vi "TX-SIS-SIM-UDP (SubVI).vi"(5 "SIS-10SDV502":bool, 6 "error in (no error)":errorcluster, 7 "SIS-10SDV501":bool, 8 "UDP Network Connection in":refnum<k16>, 9 "SIM-PC-IP":u32, 10 "SIM-PC-UDP-Port":u16, 11 "SIS-10SDV500":bool) -> (0 "UDP Network Connection out":refnum<k16>, 3 "BPCS-SIM-TX-ARRAY":i16[](array[numeric]), 4 "error out":errorcluster)   [LabVIEW 2018]
panel:
  out "length":i32[](array[numeric])
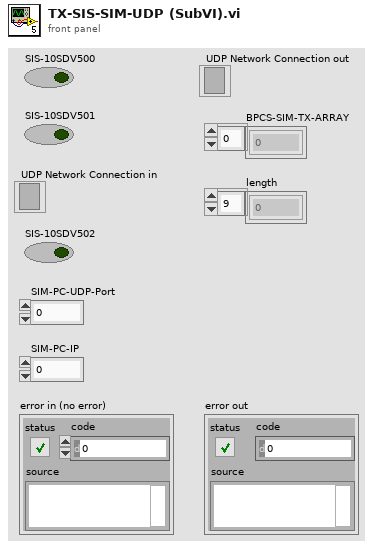
[diagram p1: front panel]
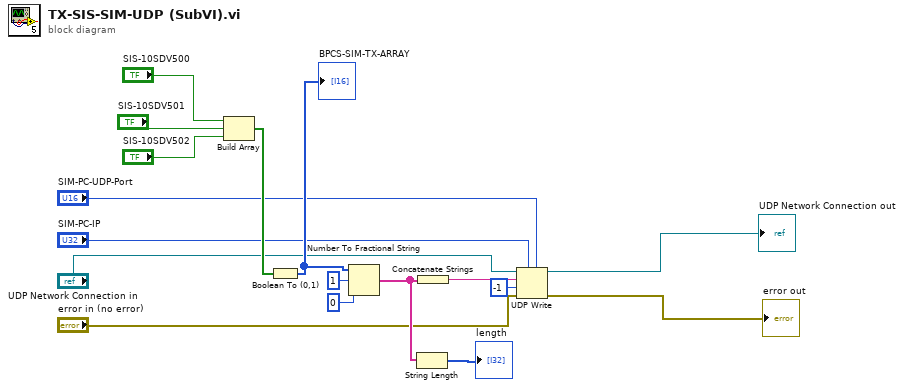
[diagram p0: block diagram]
diagram:
  n1 = Build Array("SIS-10SDV500", "SIS-10SDV501", "SIS-10SDV502") -> (w16:bool[])
  n2 = Boolean To (0,1)(Boolean=w16) -> (0, 1=w11:i16[])
  "BPCS-SIM-TX-ARRAY" <- w11
  n3 = Number To Fractional String(number=w11, width (-)=i16 1, precision (6)=i16 0) -> (F-format string=w8:string[])  [unwired: 1 in]
  n4 = String Length(string=w8) -> (length=→"length":i32[])
  n5 = Concatenate Strings(w8) -> (w1:string)
  n6 = UDP Write(address="SIM-PC-IP", port or service name="SIM-PC-UDP-Port", connection ID="UDP Network Connection in", data in=w1, 8:"error in (no error)", 9:-1 ("timeout ms (25000)")) -> (error out=→"error out":errorcluster, 3:→"UDP Network Connection out":refnum<k16>)
